vi "fillarray.vi"(3 "Numeric":dbl) -> (0 "Array":dbl[](array[numeric]))   [LabVIEW 2012]
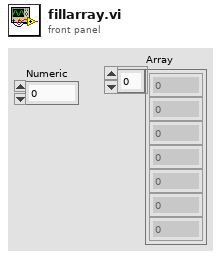
[diagram p1: front panel]
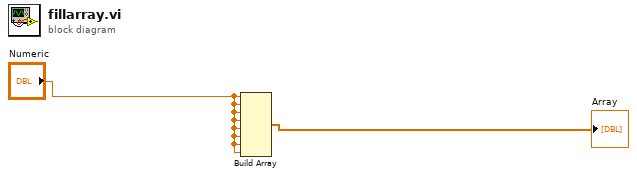
[diagram p0: block diagram]
diagram:
  n1 = Build Array("Numeric", "Numeric", "Numeric", "Numeric", "Numeric", "Numeric", "Numeric", "Numeric") -> (→"Array":dbl[])
